vi "Calculo_valores_internos.vi"(2 "todos_os_dados_ENTRADA(engenharia)":T6, 5 "todos_dados_SAIDA(controle)":T1) -> (6 "todos_dados_SAIDA":T1)   [LabVIEW 2019]
uses:
  padrao_todos_os_dados_ENTRADA.ctl
  padrao_UCM.004.EEL.0300_ENTRADA.ctl
  padrao_UCM.004.EEL.0200_ENTRADA.ctl
  padrao_INTERNO.ctl
  padrao_ADAM_ENTRADA.ctl
  padrao_todos_os_dados_SAIDA.ctl
  padrao_UCM.004.EEL.0300_SAIDA.ctl
  padrao_UCM.004.EEL.0200_SAIDA.ctl
  padrao_ADAM_SAIDA.ctl
  padrao_fluid_name_propriedades.ctl
  padrao_entry_type_propriedades.ctl
  padrao_unidades_medida_propriedades.ctl
  padrao_propriedades_propriedades.ctl
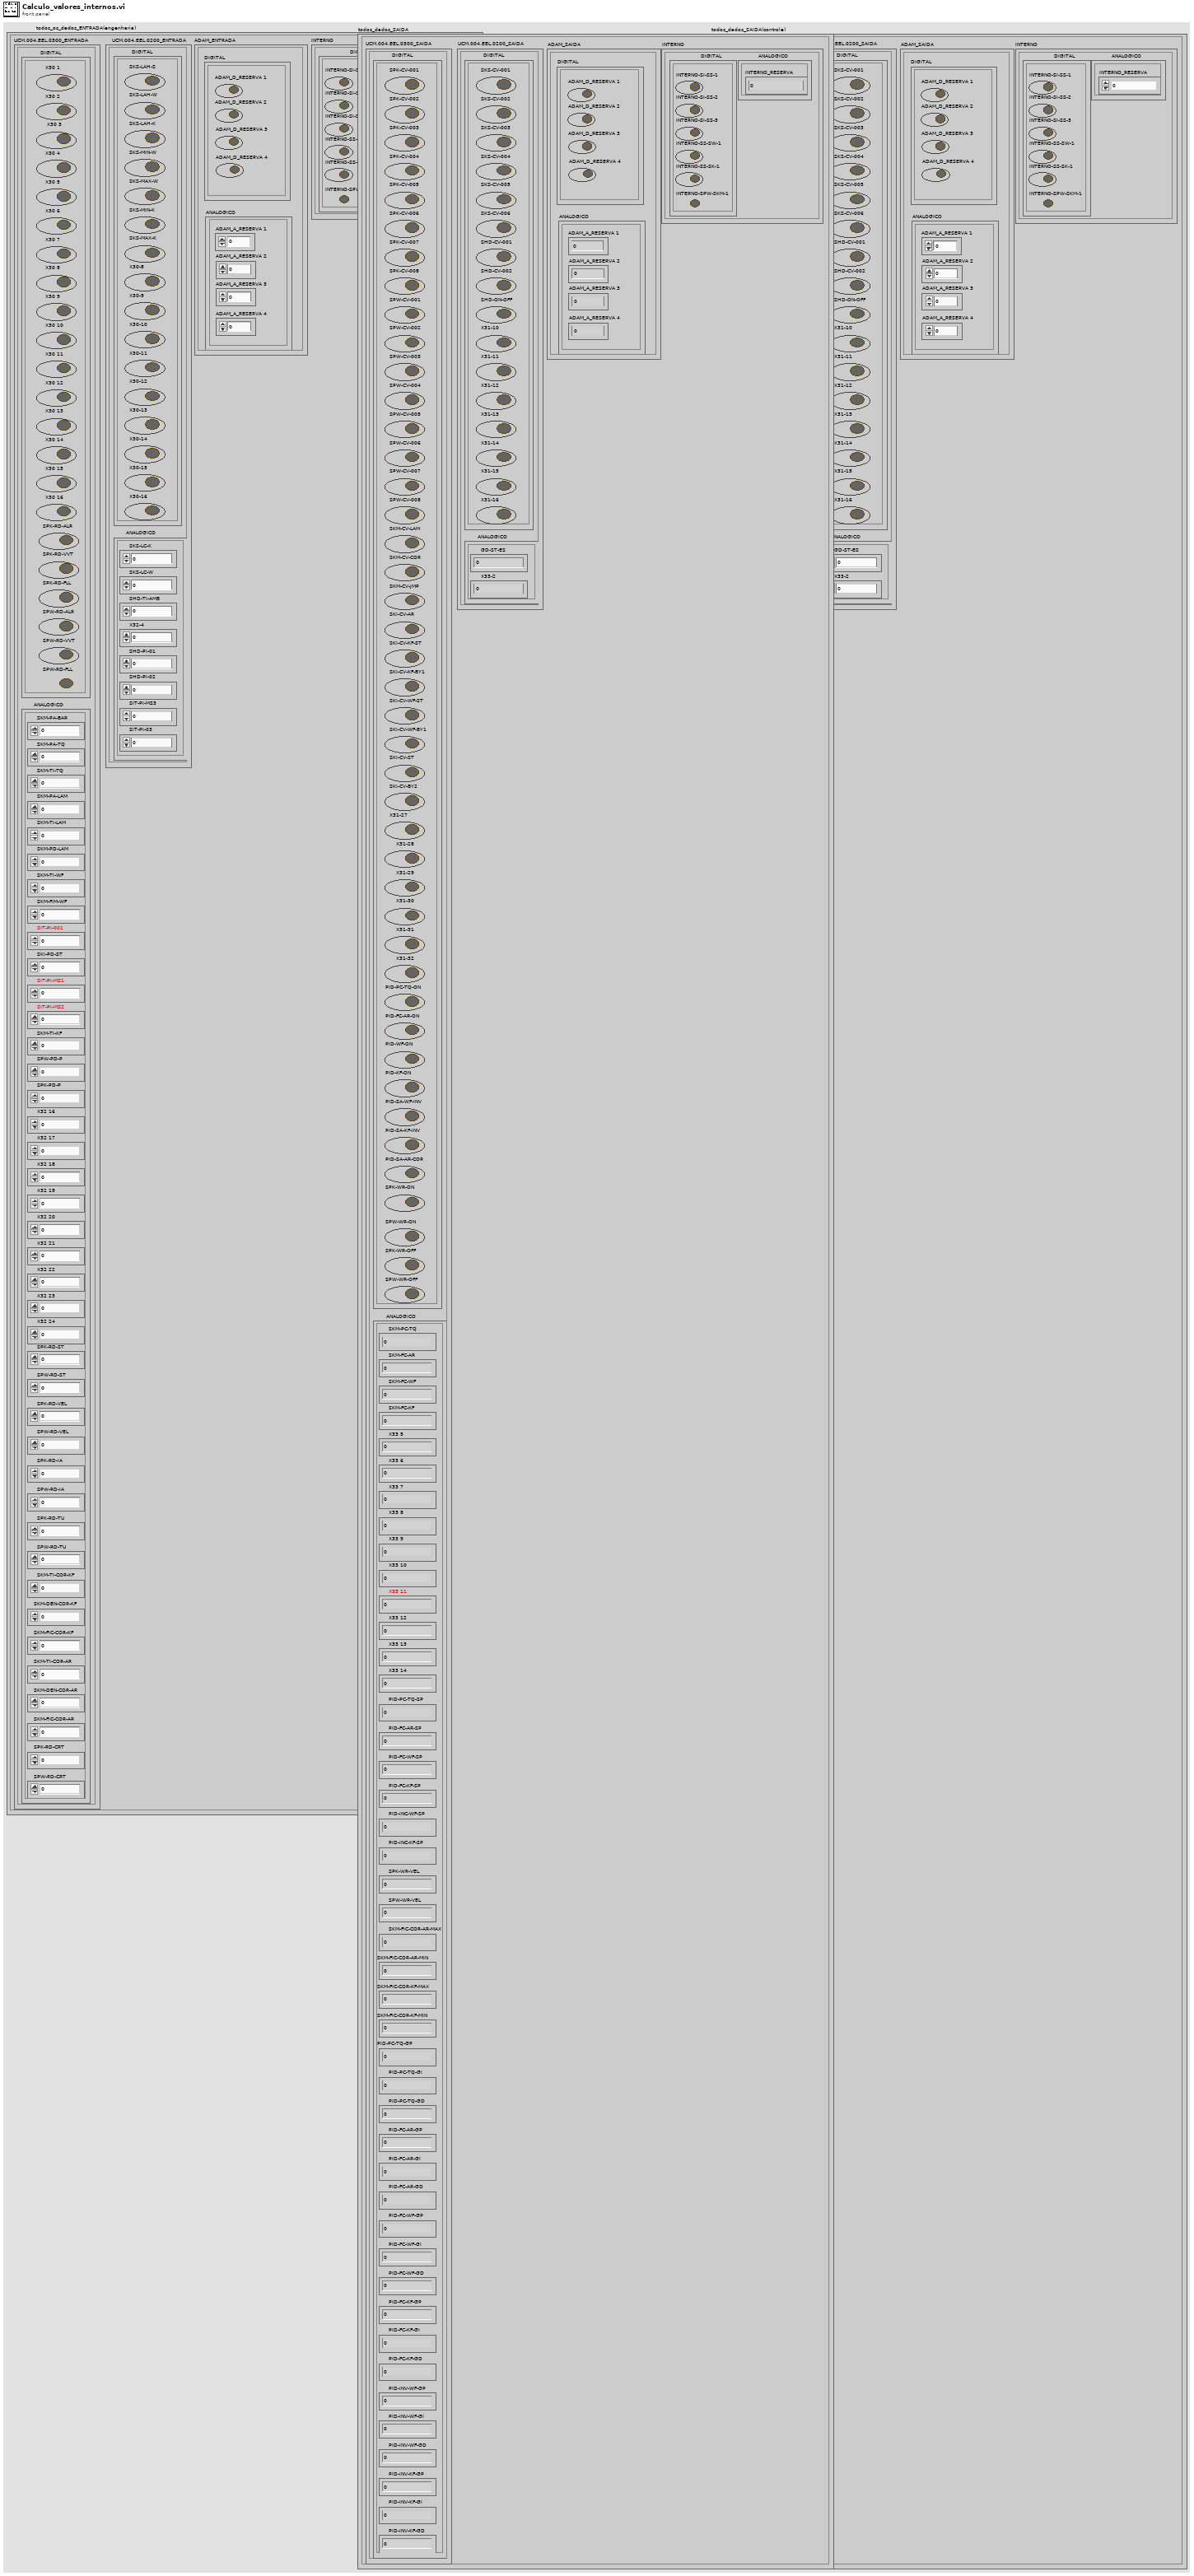
[diagram p1: front panel]
types:
  T1 = typedef "padrao_todos_os_dados_SAIDA.ctl" = cluster{"UCM.004.EEL.0300_SAIDA":T2, "UCM.004.EEL.0200_SAIDA":T3, "INTERNO":T4, "ADAM_SAIDA":T5}
  T2 = typedef "padrao_UCM.004.EEL.0300_SAIDA.ctl" = cluster{"DIGITAL":cluster{"SPK-CV-001":bool, "SPK-CV-002":bool, "SPK-CV-003":bool, "SPK-CV-004":bool, "SPK-CV-005":bool, "SPK-CV-006":bool, "SPK-CV-007":bool, "SPK-CV-008":bool, "SPW-CV-001":bool, "SPW-CV-002":bool, "SPW-CV-003":bool, "SPW-CV-004":bool, "SPW-CV-005":bool, "SPW-CV-006":bool, "SPW-CV-007":bool, "SPW-CV-008":bool, "SKM-CV-LAM":bool, "SKM-CV-COR":bool, "SKM-CV-JMP":bool, "SKI-CV-AR":bool, "SKI-CV-KF-ST":bool, "SKI-CV-KF-BY1":bool, "SKI-CV-WF-ST":bool, "SKI-CV-WF-BY1":bool, "SKI-CV-ST":bool, "SKI-CV-BY2":bool, "X31-27":bool, "X31-28":bool, "X31-29":bool, "X31-30":bool, "X31-31":bool, "X31-32":bool, "PID-PC-TQ-ON":bool, "PID-FC-AR-ON":bool, "PID-WF-ON":bool, "PID-KF-ON":bool, "PID-SA-WF-INV":bool, "PID-SA-KF-INV":bool, "PID-SA-AR-COR":bool, "SPK-WR-ON":bool, "SPW-WR-ON":bool, "SPK-WR-OFF":bool, "SPW-WR-OFF":bool}, "ANALOGICO":cluster{"SKM-PC-TQ":i16, "SKM-FC-AR":i16, "SKM-FC-WF":i16, "SKM-FC-KF":i16, "X33 5":i16, "X33 6":i16, "X33 7":i16, "X33 8":i16, "X33 9":i16, "X33 10":i16, "X33 11":i16, "X33 12":i16, "X33 13":i16, "X33 14":i16, "PID-PC-TQ-SP":i16, "PID-FC-AR-SP":i16, "PID-FC-WF-SP":i16, "PID-FC-KF-SP":i16, "PID-INC-WF-SP":i16, "PID-INC-KF-SP":i16, "SPK-WR-VEL":i32, "SPW-WR-VEL":i32, "SKM-FIC-COR-AR-MAX":dbl, "SKM-FIC-COR-AR-MIN":dbl, "SKM-FIC-COR-KF-MAX":dbl, "SKM-FIC-COR-KF-MIN":dbl, "PID-PC-TQ-GP":dbl, "PID-PC-TQ-GI":dbl, "PID-PC-TQ-GD":dbl, "PID-FC-AR-GP":dbl, "PID-FC-AR-GI":dbl, "PID-FC-AR-GD":dbl, "PID-FC-WF-GP":dbl, "PID-FC-WF-GI":dbl, "PID-FC-WF-GD":dbl, "PID-FC-KF-GP":dbl, "PID-FC-KF-GI":dbl, "PID-FC-KF-GD":dbl, "PID-INV-WF-GP":dbl, "PID-INV-WF-GI":dbl, "PID-INV-WF-GD":dbl, "PID-INV-KF-GP":dbl, "PID-INV-KF-GI":dbl, "PID-INV-KF-GD":dbl}}
  T3 = typedef "padrao_UCM.004.EEL.0200_SAIDA.ctl" = cluster{"DIGITAL":cluster{"SKS-CV-001":bool, "SKS-CV-002":bool, "SKS-CV-003":bool, "SKS-CV-004":bool, "SKS-CV-005":bool, "SKS-CV-006":bool, "SHD-CV-001":bool, "SHD-CV-002":bool, "SHD-ON-OFF":bool, "X31-10":bool, "X31-11":bool, "X31-12":bool, "X31-13":bool, "X31-14":bool, "X31-15":bool, "X31-16":bool}, "ANALOGICO":cluster{"GD-ST-ES":i16, "X33-2":i16}}
  T4 = typedef "padrao_INTERNO.ctl" = cluster{"DIGITAL":cluster{"INTERNO-SI-SS-1":bool, "INTERNO-SI-SS-2":bool, "INTERNO-SI-SS-3":bool, "INTERNO-SS-SW-1":bool, "INTERNO-SS-SK-1":bool, "INTERNO-SPW-SKM-1":bool}, "ANALOGICO":cluster{"INTERNO_RESERVA":dbl}}
  T5 = typedef "padrao_ADAM_SAIDA.ctl" = cluster{"DIGITAL":cluster{"ADAM_D_RESERVA 1":bool, "ADAM_D_RESERVA 2":bool, "ADAM_D_RESERVA 3":bool, "ADAM_D_RESERVA 4":bool}, "ANALOGICO":cluster{"ADAM_A_RESERVA 1":dbl, "ADAM_A_RESERVA 2":dbl, "ADAM_A_RESERVA 3":dbl, "ADAM_A_RESERVA 4":dbl}}
  T6 = typedef "padrao_todos_os_dados_ENTRADA.ctl" = cluster{"UCM.004.EEL.0300_ENTRADA":T7, "UCM.004.EEL.0200_ENTRADA":T8, "INTERNO":T4, "ADAM_ENTRADA":T9}
  T7 = typedef "padrao_UCM.004.EEL.0300_ENTRADA.ctl" = cluster{"DIGITAL":cluster{"X30 1":bool, "X30 2":bool, "X30 3":bool, "X30 4":bool, "X30 5":bool, "X30 6":bool, "X30 7":bool, "X30 8":bool, "X30 9":bool, "X30 10":bool, "X30 11":bool, "X30 12":bool, "X30 13":bool, "X30 14":bool, "X30 15":bool, "X30 16":bool, "SPK-RD-ALR":bool, "SPK-RD-VVT":bool, "SPK-RD-FLL":bool, "SPW-RD-ALR":bool, "SPW-RD-VVT":bool, "SPW-RD-FLL":bool}, "ANALOGICO":cluster{"SKM-PA-BAR":i16, "SKM-PA-TQ":i16, "SKM-TI-TQ":i16, "SKM-PA-LAM":i16, "SKM-TI-LAM":i16, "SKM-PD-LAM":i16, "SKM-TI-WF":i16, "SKM-FIM-WF":i16, "SIT-PI-001":i16, "SKI-PD-ST":i16, "SIT-PI-MS1":i16, "SIT-PI-MS2":i16, "SKM-TI-KF":i16, "SPW-PD-P":i16, "SPK-PD-P":i16, "X32 16 ":i16, "X32 17":i16, "X32 18":i16, "X32 19":i16, "X32 20":i16, "X32 21":i16, "X32 22":i16, "X32 23":i16, "X32 24":i16, "SPK-RD-ST":i32, "SPW-RD-ST":i32, "SPK-RD-VEL":i32, "SPW-RD-VEL":i32, "SPK-RD-IA":i32, "SPW-RD-IA":i32, "SPK-RD-TU":i32, "SPW-RD-TU":i32, "SKM-TI-COR-KF":dbl, "SKM-DEN-COR-KF":dbl, "SKM-FIC-COR-KF":dbl, "SKM-TI-COR-AR":dbl, "SKM-DEN-COR-AR":dbl, "SPK-RD-CRT":dbl, "SPW-RD-CRT":dbl, "SKM-FIC-COR-AR":dbl}}
  T8 = typedef "padrao_UCM.004.EEL.0200_ENTRADA.ctl" = cluster{"DIGITAL":cluster{"SKS-LAH-S":bool, "SKS-LAH-W":bool, "SKS-LAH-K":bool, "SKS-MIN-W":bool, "SKS-MAX-W":bool, "SKS-MIN-K":bool, "SKS-MAX-K":bool, "X30-8":bool, "X30-9":bool, "X30-10":bool, "X30-11":bool, "X30-12":bool, "X30-13":bool, "X30-14":bool, "X30-15":bool, "X30-16":bool}, "ANALOGICO":cluster{"SKS-LC-K":i16, "SKS-LC-W":i16, "SHD-TI-AMB":i16, "X32-4":i16, "SHD-PI-01":i16, "SHD-PI-02":i16, "SIT-PI-MS3":i16, "SIT-PI-03":i16}}
  T9 = typedef "padrao_ADAM_ENTRADA.ctl" = cluster{"DIGITAL":cluster{"ADAM_D_RESERVA 1":bool, "ADAM_D_RESERVA 2":bool, "ADAM_D_RESERVA 3":bool, "ADAM_D_RESERVA 4":bool}, "ANALOGICO":cluster{"ADAM_A_RESERVA 1":dbl, "ADAM_A_RESERVA 2":dbl, "ADAM_A_RESERVA 3":dbl, "ADAM_A_RESERVA 4":dbl}}
  T10 = typedef "padrao_propriedades_propriedades.ctl" = string
  T11 = typedef "padrao_unidades_medida_propriedades.ctl" = string
  T12 = typedef "padrao_entry_type_propriedades.ctl" = string
  T13 = typedef "padrao_fluid_name_propriedades.ctl" = string
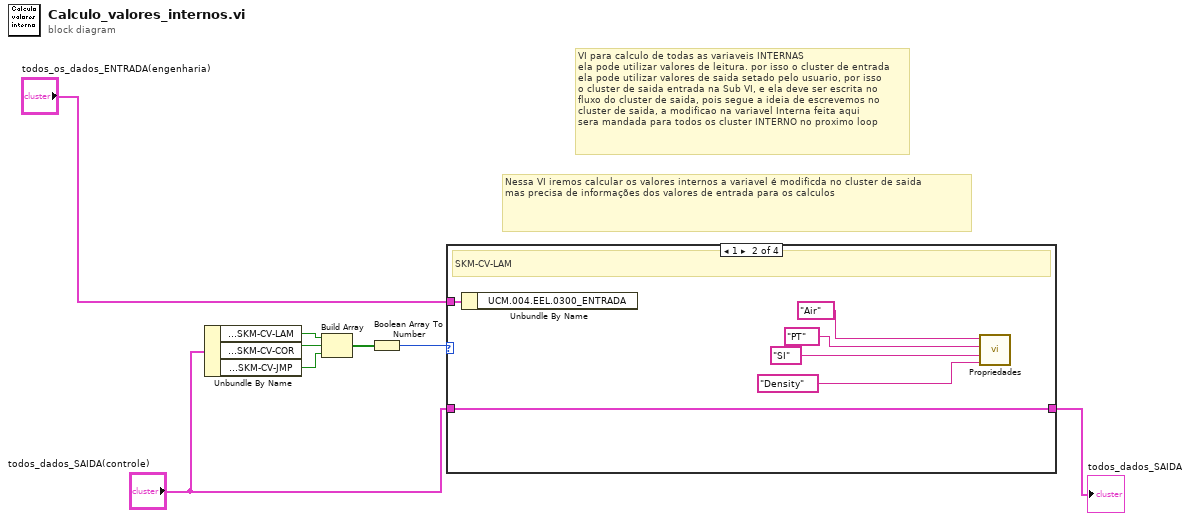
[diagram p0: block diagram]
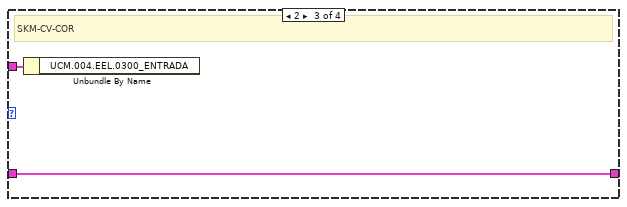
[diagram p3: hidden frame]
diagram:
  # "VI para calculo de todas as variaveis INTERNAS\nela pode utilizar valores de leitura. por isso o cluster de entrada\nela pode utilizar valores de saida setado pelo usuario, por isso\no cluster de saida entrada na Sub VI, e ela deve ser escrita no\nfluxo do cluster de saida, pois segue a ideia de escrevemos no\ncluster de saida, a modificao na variavel Interna feita aqui \nsera mandada para todos os cluster INTERNO no proximo loop"
  # "Nessa VI iremos calcular os valores internos a variavel é modificda no cluster de saida\nmas precisa de informações dos valores de entrada para os calculos"
  n1 = Unbundle By Name("todos_dados_SAIDA(controle)") -> ("UCM.004.EEL.0300_SAIDA.DIGITAL.SKM-CV-LAM"=w7:bool, "UCM.004.EEL.0300_SAIDA.DIGITAL.SKM-CV-COR"=w6:bool, "UCM.004.EEL.0300_SAIDA.DIGITAL.SKM-CV-JMP"=w1:bool)
  n2 = Build Array(w7, w6, w1) -> (w5:bool[])
  n3 = Boolean Array To Number(Boolean array=w5) -> (number=w4:u32)
  n4 = case shown="1" w4 {
    tunnel: "todos_os_dados_ENTRADA(engenharia)" -> [_ w15 w17 _]
    tunnel: [w9 w14 w16 w18] -> w3
    tunnel: "todos_dados_SAIDA(controle)" -> [w9 w14 w16 w18]
    frame 0, Default {
      # "Nenhum caminho aberto para calculo"
    }
    frame 1 {
      # "SKM-CV-LAM"
      n5 = Unbundle By Name(w15) -> ()  [unwired: 1 out]
      n6 = call "Propriedades.vi"("Propriedades"=T10 "Density", "Unidade"=T11 "SI", "Entry Type"=T12 "PT", "Fluid Name"=T13 "Air") -> ()  [unwired: 4 in, 1 out]
    }
    frame 2 {
      # "SKM-CV-COR"
      n7 = Unbundle By Name(w17) -> ()  [unwired: 1 out]
    }
    frame 3 {
      # "SKM-CV-LAM & SKM-CV-COR Abertos, indicar erro\nNAN"
    }
  }
  "todos_dados_SAIDA" <- w3
